vi "Plot Frequency Response.vi"   [LabVIEW 2016]
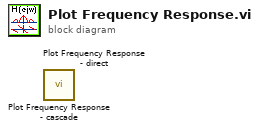
[diagram p0: block diagram]
diagram:
  n1 = call "Plot Frequency Response - cascade.vi"() -> ()  [unwired: 5 in, 3 out]
  n2 = call "Plot Frequency Response - direct.vi"() -> ()  [unwired: 5 in, 3 out]
